vi "Read Trace data mMc.vi"(1 "Port":T1={"P type"=0, "reference"="", " Terminator "="\r\n", "Timeout"=300} {"Timeout" step=10; "P type" items=["none", "RS-232C"]}, 3 "error in (no error)":errorcluster, 5 "Controller #":string) -> (6 "# samples":i32, 7 "Tr data":string, 9 "error out":errorcluster)   [LabVIEW 2011]
uses:
  mMc - global.vi
panel:
  # "Read Trace data"
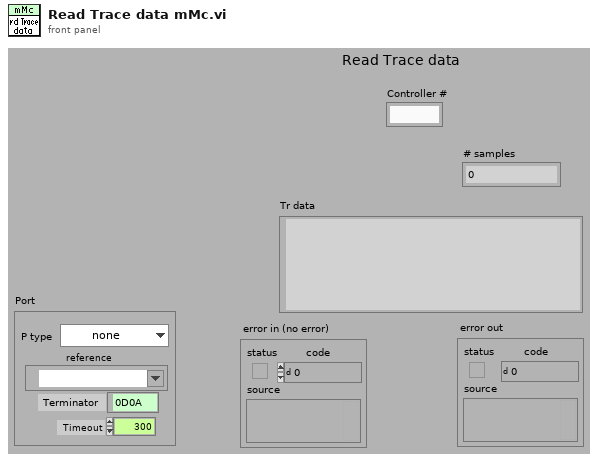
[diagram p1: front panel]
types:
  T1 = cluster{"P type":u16, "reference":refnum<visa-resource-name>, " Terminator ":string, "Timeout":i32}
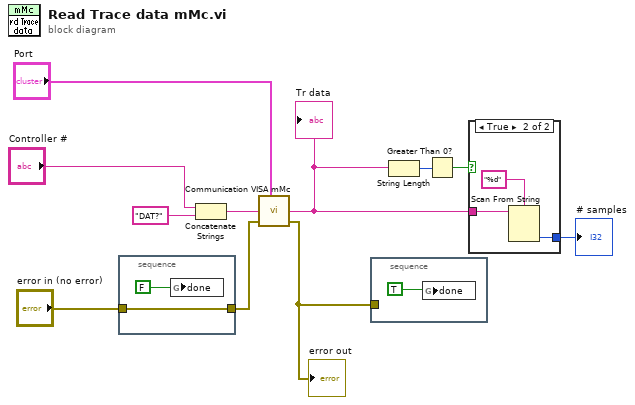
[diagram p0: block diagram]
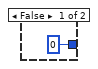
[diagram p2: hidden frame]
diagram:
  n1 = stacked-sequence {
    tunnel: "error in (no error)" -> [w13]
    tunnel: [w13] -> w5
    frame #0 {
      n2 = global write "mMc - global.vi" "done"(FALSE ("done")) -> ()
    }
  }
  n3 = Concatenate Strings("Controller #", "DAT?") -> (w8:string)
  n4 = call "Communication VISA mMc.vi"("Port"="Port", "Command"=w8, "error in (no error)"=w5) -> ("Return"=w3:string, "error out"=w4:errorcluster)  [unwired: 3 in, 2 out]
  "error out" <- w4
  "Tr data" <- w3
  n5 = stacked-sequence {
    tunnel: w4 -> [_]
    frame #0 {
      n6 = global write "mMc - global.vi" "done"(TRUE ("done")) -> ()
    }
  }
  n7 = String Length(string=w3) -> (length=w2:i32)
  n8 = Greater Than 0?(x=w2) -> (x > 0?=w1:bool)
  n9 = case shown="True" w1 {
    tunnel: [0 w18] -> w7
    tunnel: w3 -> [_ w17]
    frame False {
    }
    frame True {
      n10 = Scan From String(format string="%d", input string=w17) -> (output 1=w18:i32)  [unwired: 3 in, 3 out]
    }
  }
  "# samples" <- w7
